vi "GOOP_CheckClassFolder.vi"(11 "Class Or Class Floder":path) -> (0 "ClassFolder":bool, 1 "FileExists":bool, 2 "Directory":bool, 3 "ClassFolder":path, 4 "ClassPath":path)   [LabVIEW 2020, in "ClassWriterGOOP300.lvclass"]
uses:
  <resource>/Framework/Providers/Open_GDS/ClassProviders/Provider_EndevoGOOP300/ClassWriterGOOP300_class/ClassWriterGOOP300.lvclass
  <vilib>/Utility/lvfile.llb/NI_FileType.lvlib
  <vilib>/Utility/LVLibp/NI_PackedLibraryUtility.lvlib
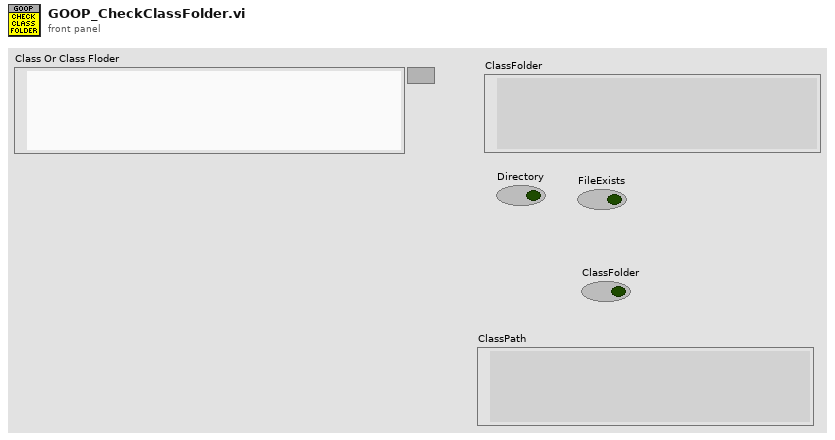
[diagram p1: front panel]
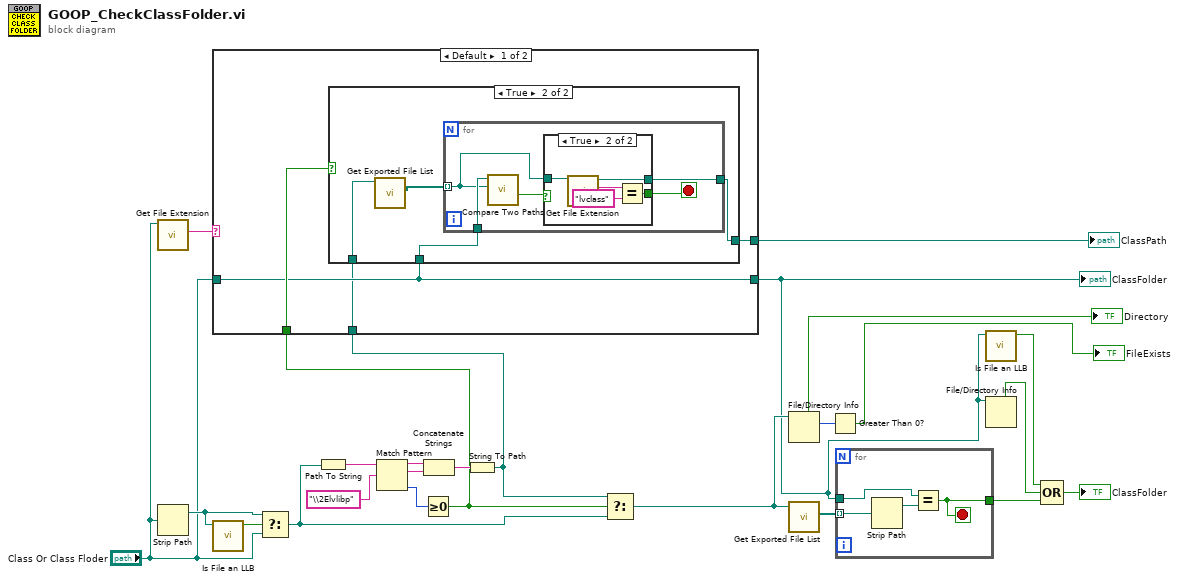
[diagram p0: block diagram]
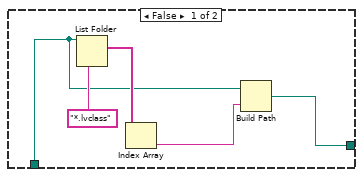
[diagram p2: hidden frame]
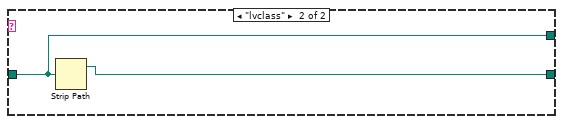
[diagram p4: hidden frame]
diagram:
  n1 = call <vilib>:"Get File Extension.vi"("file"="Class Or Class Floder") -> ("lowercase file extension"=w7:string)  [unwired: 6 in, 4 out]
  n2 = Strip Path(path="Class Or Class Floder") -> (stripped path=w24:path)  [unwired: 1 out]
  n3 = call <vilib>:"Is File an LLB.vi"("path"=w24) -> ("Is LLB?"=w23:bool)  [unwired: 9 in, 1 out]
  n4 = Select(t=w24, s=w23, f="Class Or Class Floder") -> (s? t:f=w14:path)
  n5 = Path To String(path=w14) -> (string=w20:string)
  n6 = Match Pattern(string=w20, regular expression="\\2Elvlibp") -> (before substring=w17:string, match substring=w16:string, offset past match=w18:i32)  [unwired: 1 in, 1 out]
  n7 = Greater Or Equal To 0?(x=w18) -> (x >= 0?=w2:bool)
  n8 = Concatenate Strings(w17, w16) -> (w15:string)
  n9 = String To Path(string=w15) -> (path=w1:path)
  n10 = case shown="Default" w7 {
    tunnel: [w27 w49] -> w3
    tunnel: "Class Or Class Floder" -> [w27 w48]
    tunnel: [w26 w48] -> w6
    tunnel: w2 -> [w28 _]
    tunnel: w1 -> [w25 _]
    frame Default {
      n11 = case shown="True" w28 {
        tunnel: w27 -> [w30 w35]
        tunnel: [w29 w34] -> w26
        tunnel: w25 -> [_ w37]
        frame False {
          n12 = List Folder(path=w30, pattern="*.lvclass" ("string")) -> (filenames=w32:string[])  [unwired: 2 in, 3 out]
          n13 = Index Array(array=w32) -> (element=w31:string)  [unwired: 1 in]
          n14 = Build Path(base path=w30, name or relative path=w31) -> (appended path=w29:path)
        }
        frame True {
          n15 = call <vilib>:"Get Exported File List.vi"("packed library path"=w37) -> ("paths"=w36:path[])  [unwired: 8 in, 2 out]
          n16 = for {
            tunnel: w36 -> [w38] mode=indexing
            tunnel: w35 -> [w42]
            tunnel: [w39] -> w34
            stop <- w40 stop-if-true
            n17 = call <vilib>:"Compare Two Paths.vi"("Path 2"=w38, "Path 1"=w42) -> ("Path 2 Relative to Path 1?"=w41:bool)  [unwired: 6 in, 3 out]
            n18 = case shown="True" w41 {
              tunnel: w38 -> [_ w47]
              tunnel: [_ w44] -> w40
              tunnel: [_ w43] -> w39
              frame False {
              }
              frame True {
                n19 = call <vilib>:"Get File Extension.vi"("file"=w47) -> ("lowercase file extension"=w46:string, "dup file"=w43:path)  [unwired: 6 in, 3 out]
                n20 = Equal?(x=w46, y="lvclass") -> (x = y?=w44:bool)
              }
            }
          }
        }
      }
    }
    frame "lvclass" {
      n21 = Strip Path(path=w48) -> (stripped path=w49:path)  [unwired: 1 out]
    }
  }
  "ClassFolder" <- w3
  "ClassPath" <- w6
  n22 = Select(t=w1, s=w2, f=w14) -> (s? t:f=w10:path)
  n23 = File/Directory Info(path=w10) -> (directory=→"Directory":bool, size=w21:i64)  [unwired: 1 in, 5 out]
  n24 = call <vilib>:"Get Exported File List.vi"("packed library path"=w10) -> ("paths"=w9:path[])  [unwired: 8 in, 2 out]
  n25 = Greater Than 0?(x=w21) -> (x > 0?=→"FileExists":bool)
  n26 = for {
    tunnel: w9 -> [w53] mode=indexing
    tunnel: w3 -> [w51]
    tunnel: [w50] -> w8
    stop <- w50 stop-if-true
    n27 = Strip Path(path=w53) -> (stripped path=w52:path)  [unwired: 1 out]
    n28 = Equal?(x=w51, y=w52) -> (x = y?=w50:bool)
  }
  n29 = call <vilib>:"Is File an LLB.vi"("path"=w3) -> ("Is LLB?"=w12:bool)  [unwired: 9 in, 1 out]
  n30 = File/Directory Info(path=w3) -> (directory=w13:bool)  [unwired: 1 in, 6 out]
  n31 = Compound Arithmetic op=OR(w12, w13, w8) -> (→"ClassFolder":bool)
